vi "Fast IV Contour vs Time.vi"(8 "error in":errorcluster, 11 "Book number":i32=335) -> (0 "error out":errorcluster)   [LabVIEW 2021]
uses:
  global.vi
  <vilib>/Utility/file.llb/Write Delimited Spreadsheet (DBL).vi
panel:
  in  "Agi Address":string="GPIB0::10::INSTR"
  in  "SRS resource name":string
  in  "Pre V Scale factor":dbl=0.0005
  in  "stop":bool
  out "Time till next scan":i32=1
  in  "Wait per scan s":i32=600
  in  "Agi T or SRS F":bool=TRUE
  in  "Average times":i32=20
  in  "Current step uA":dbl=0.004 format="%#_13g"
  in  "Voltage Read  channel":tag="Dev1/ai1"
  in  "samples per channel":i32=2000
  in  "Trigger source":tag="/Dev1/PFI12"
  in  "DAQ rate":dbl=100000.0 format="%#_13g"
  in  "Frequency Hz":dbl=50.0
  in  "Vmax":dbl=4.0
  in  "Contour plot folder":path=path "\\\\ad.uillinois.edu\\engr/mrl-dvh-research/Guang Yue/data/Contour plot"
  # "Check DAQ fast IV.vi to set default values ex scale factor etc."
  # "Scale * Vread=Vdevice"
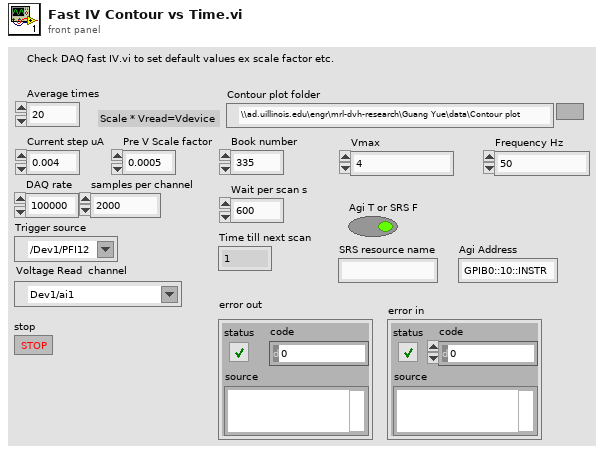
[diagram p1: front panel]
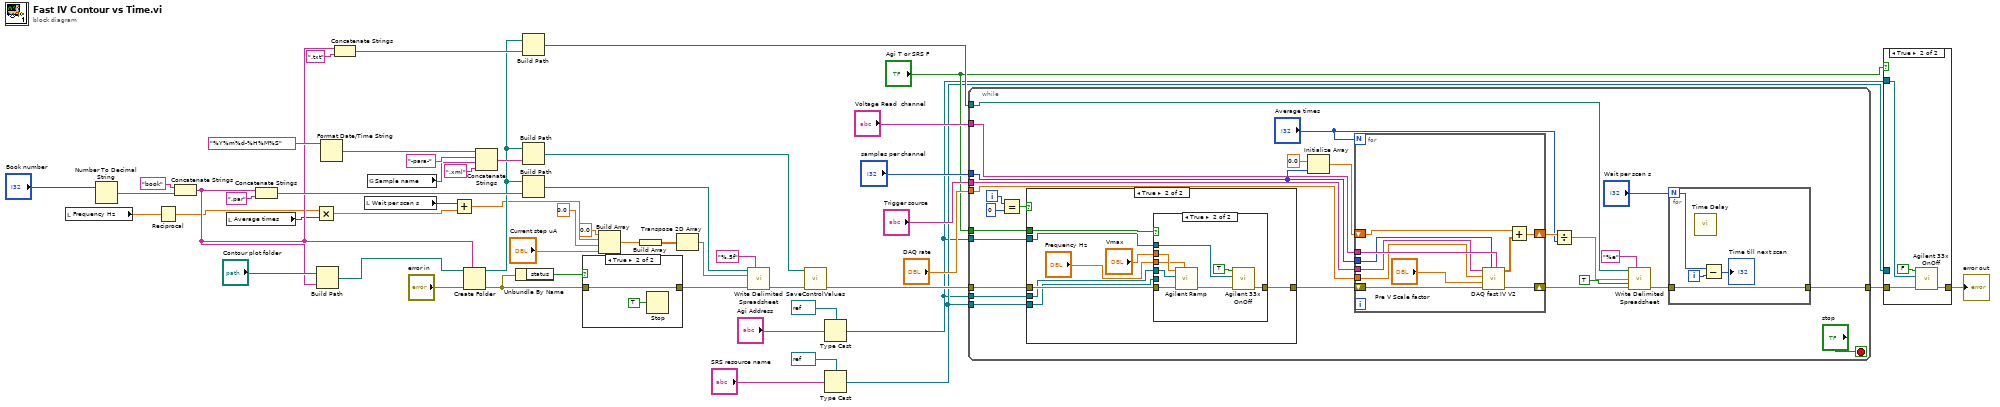
[diagram p0: block diagram]
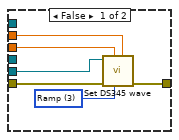
[diagram p3: hidden frame]
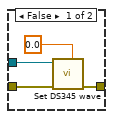
[diagram p4: hidden frame]
diagram:
  n1 = local read "Frequency Hz"() -> (w12:dbl)
  n2 = Number To Decimal String(number="Book number") -> (decimal integer string=w18:string)  [unwired: 1 in]
  n3 = Reciprocal(x=w12) -> (1/x=w11:dbl)
  n4 = Concatenate Strings("book" ("string"), w18) -> (w16:string)
  n5 = local read "Average times"() -> (w10:i32)
  n6 = Concatenate Strings(w16, ".par" ("string")) -> (w45:string)
  n7 = Multiply(x=w11, y=w10) -> (x*y=w9:dbl)
  n8 = Build Path(base path="Contour plot folder", name or relative path=w16) -> (appended path=w35:path)
  n9 = Format Date/Time String(time format string (%c)="%Y%m%d-%H%M%S") -> (date/time string=w29:string)  [unwired: 2 in]
  n10 = Concatenate Strings(w16, ".txt" ("string")) -> (w38:string)
  n11 = local read "Wait per scan s"() -> (w13:i32)
  n12 = global read "global.vi" "Sample name"() -> (w28:string)
  n13 = Add(x=w13, y=w9) -> (x+y=w8:dbl)
  n14 = Create Folder(prompt (Create Folder)=w16, path (use dialog)=w35, error in="error in") -> (created path=w30:path, error out=w32:errorcluster)  [unwired: 1 out]
  n15 = Concatenate Strings(w29, "-para-" ("string"), w28, ".xml" ("string")) -> (w49:string)
  n16 = Unbundle By Name(w32) -> ("status"=w33:bool)
  n17 = Build Path(base path=w30, name or relative path=w38) -> (appended path=w37:path)
  n18 = Build Path(base path=w30, name or relative path=w49) -> (appended path=w47:path)
  n19 = Build Path(base path=w30, name or relative path=w45) -> (appended path=w44:path)
  n20 = case shown="True" w33 {
    tunnel: [w53 w55] -> w31
    tunnel: w32 -> [w53 w55]
    frame False {
    }
    frame True {
      n21 = Stop(stop? (T)=TRUE) -> ()
    }
  }
  n22 = Build Array(0.0 ("element"), w8, 0.0 ("element"), "Current step uA") -> (w42:dbl[])
  n23 = Build Array(w42) -> (w41:dbl[][])
  n24 = Transpose 2D Array(2D array=w41) -> (transposed array=w40:dbl[][])
  n25 = call-poly <vilib>:"Write Delimited Spreadsheet.vi"("file path (dialog if empty)"=w44, "format (%.3f)"="%.5f", "2D data"=w40, "error in (no error)"=w31) -> ("error out"=w34:errorcluster)  [unwired: 10 in, 1 out]
  n26 = call "SaveControlValues.vi"("XML File Path"=w47, "error in (no error)"=w34) -> ("error out"=w27:errorcluster)  [unwired: 8 in]
  n27 = Type Cast(type=refnum<visa-resource-name> refnum ("SRS resource name 2"), x="Agi Address") -> (*(type *) &x=w1:refnum<visa-resource-name>)
  n28 = Type Cast(type=refnum<visa-resource-name> refnum ("SRS resource name 2"), x="SRS resource name") -> (*(type *) &x=w2:refnum<visa-resource-name>)
  n29 = while {
    tunnel: w37 -> [w77]
    tunnel: w27 -> [w75]
    tunnel: [w61] -> w14
    tunnel: "Voltage Read  channel" -> [w72]
    tunnel: "samples per channel" -> [w65]
    tunnel: "Trigger source" -> [w71]
    tunnel: "DAQ rate" -> [w70]
    tunnel: "Agi T or SRS F" -> [w63]
    tunnel: w2 -> [w58]
    tunnel: w1 -> [w57]
    tunnel: w1 -> [w56]
    i -> [w81]
    stop <- "stop" stop-if-true
    n30 = Equal?(x=w81, y=0) -> (x = y?=w76:bool)
    n31 = case shown="True" w76 {
      tunnel: w75 -> [w96 w100]
      tunnel: [w96 w104] -> w74
      tunnel: w63 -> [_ w103]
      tunnel: w58 -> [_ w99]
      tunnel: w57 -> [_ w98]
      tunnel: w56 -> [_ w97]
      frame False {
      }
      frame True {
        n32 = case shown="True" w103 {
          tunnel: [w108 w117] -> w104
          tunnel: "Vmax" -> [w107 w115]
          tunnel: "Frequency Hz" -> [w106 w114]
          tunnel: w100 -> [w109 w113]
          tunnel: w99 -> [w105 _]
          tunnel: w98 -> [_ w112]
          tunnel: w97 -> [_ w111]
          frame False {
            w110 = u16 3 items=["Sine", "Square", "Triangle", "Ramp", "Noise"] ("Waveform Function (0: Sine)")
            n33 = call "Set DS345 wave.vi"("Amplitude (0.01 Vpp)"=w107, "Waveform Function (0: Sine)"=w110, "Frequency (1000 Hz)"=w106, "error in (no error)"=w109, "VISA resource name"=w105) -> ("error out"=w108:errorcluster)  [unwired: 6 in]
          }
          frame True {
            n34 = call "Agilent Ramp.vi"("Frequency Hz"=w114, "error in (no error)"=w113, "VISA resource name"=w112, "Vmax"=w115) -> ("error out"=w118:errorcluster)  [unwired: 7 in]
            n35 = call "Agilent 33x OnOff.vi"("error in (no error)"=w118, "VISA resource name"=w111, "Enable Output  (T: Enable)"=TRUE) -> ("error out"=w117:errorcluster)  [unwired: 8 in]
          }
        }
      }
    }
    n36 = Initialize Array(0.0 ("element"), w65) -> (w64:dbl[])
    n37 = for {
      N: "Average times" -> [_]
      tunnel: w72 -> [w93]
      tunnel: w65 -> [w92]
      tunnel: w71 -> [w91]
      tunnel: w70 -> [w90]
      shift-right: [w94] -> w73
      shift-left: w74 -> [w95]
      shift-right: [w88] -> w69
      shift-left: w64 -> [w87]
      n38 = call "DAQ fast IV V2.vi"("physical channels I and V"=w93, "samples per channel"=w92, "error in"=w95, 9:"Pre V Scale factor", "rate"=w90, "Trigger source"=w91) -> ("error out"=w94:errorcluster, "Output"=w89:dbl[][])  [unwired: 4 in]
      n39 = Add(x=w87, y=w89) -> (x+y=w88:dbl[])
    }
    n40 = Divide(x=w69, y="Average times") -> (x/y=w67:dbl[])
    n41 = call-poly <vilib>:"Write Delimited Spreadsheet.vi"("file path (dialog if empty)"=w77, "format (%.3f)"="%e", "1D data"=w67, "append to file? (new file:F)"=TRUE ("append to file? (F)"), "error in (no error)"=w73) -> ("error out"=w62:errorcluster)  [unwired: 9 in, 1 out]
    n42 = for {
      N: "Wait per scan s" -> [w84]
      tunnel: [w85] -> w61
      tunnel: w62 -> [w85]
      i -> [w83]
      n43 = call "Time Delay"() -> ()  [unwired: 11 in, 1 out]
      n44 = Subtract(x=w84, y=w83) -> (x-y=→"Time till next scan":i32)
    }
  }
  n45 = case shown="True" "Agi T or SRS F" {
    tunnel: w14 -> [w122 w126]
    tunnel: [w121 w125] -> w26
    tunnel: w2 -> [w119 _]
    tunnel: w1 -> [_ w123]
    frame False {
      n46 = call "Set DS345 wave.vi"("Amplitude (0.01 Vpp)"=0.0, "error in (no error)"=w122, "VISA resource name"=w119) -> ("error out"=w121:errorcluster)  [unwired: 8 in]
    }
    frame True {
      n47 = call "Agilent 33x OnOff.vi"("error in (no error)"=w126, "VISA resource name"=w123, "Enable Output  (T: Enable)"=FALSE) -> ("error out"=w125:errorcluster)  [unwired: 8 in]
    }
  }
  "error out" <- w26
